vi "FTW-Regex-CapturingGroups.vi"(0 "Regex":refnum<data-value>, 11 "error in":errorcluster) -> (4 "Regex out":refnum<data-value>, 6 "Capture Groups":string[](array[string]), 15 "error out":errorcluster)   [LabVIEW 2014]
uses:
  core/FTW-Regex-Core-Structure.ctl
  error/FTW-ERR-ThrowError.vi
  error/FTW-ERR-NoErrorConstant.vi
  error/FTW-ERR-CallChain.vi
  string/FTW-STR-ReplaceWhitespace.vi
panel:
  # "Inputs"
  # "Outputs"
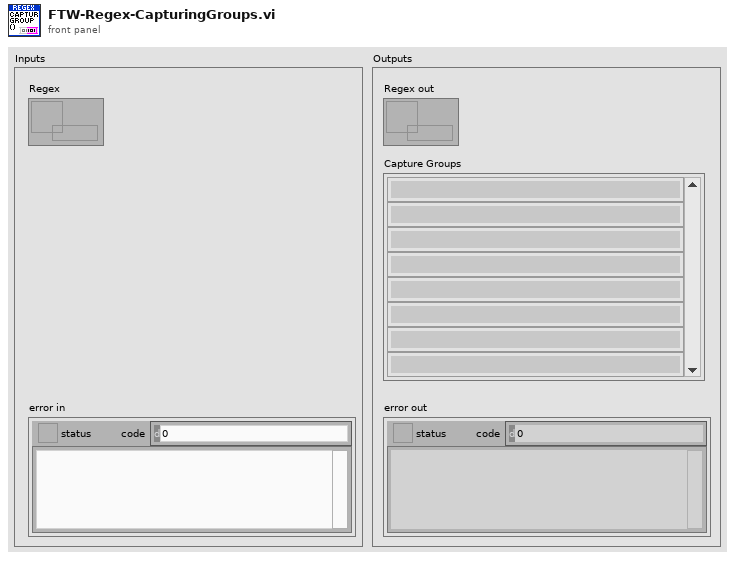
[diagram p1: front panel]
types:
  T1 = typedef "FTW-Regex-Core-Structure.ctl" = cluster{"Compiled Regex":u64}
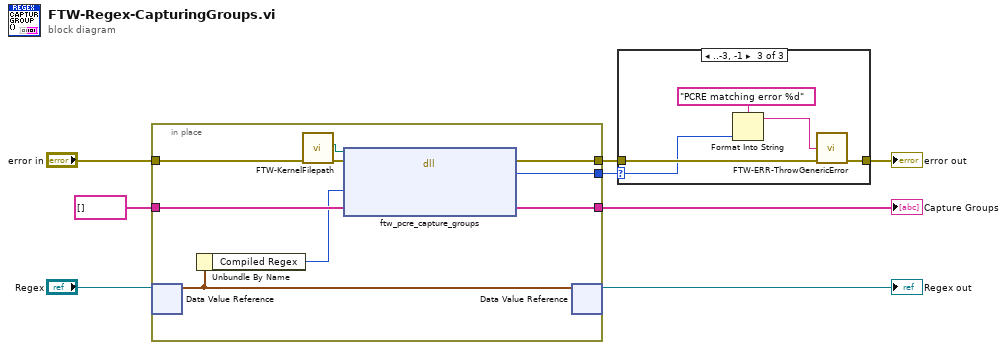
[diagram p0: block diagram]
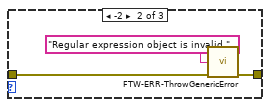
[diagram p3: hidden frame]
diagram:
  n1 = in-place {
    in-place-border: [w17] -> w5
    in-place-border: "error in" -> [w11]
    in-place-border: [w16] -> w7
    in-place-border: [w15] -> w4
    in-place-border: string[] [] -> [w14]
    n2 = in-place-dvr #1("Regex") -> (w13:T1)  [unwired: 1 out]
    n3 = Unbundle By Name(w13) -> ("Compiled Regex"=w12:u64)
    n4 = call "FTW-KernelFilepath.vi"("error in"=w11) -> ("error out"=w10:errorcluster, "Library Filepath"=w9:path)  [unwired: 8 in, 1 out]
    n5 = dll-call lib="?" fn="ftw_pcre_capture_groups"(path in=w9, error in=w10, "Compiled Regex"=w12, "Capture Groups"=w14) -> (error out=w17:errorcluster, "Return Value"=w16:i64, "Capture Groups"=w15:string[])  [unwired: 2 in, 1 out]
    n6 = in-place-dvr #1(w13) -> (→"Regex out":refnum<data-value>)  [unwired: 1 out]
  }
  "Capture Groups" <- w4
  n7 = case shown="..-3, -1" w7 {
    selector: w7 -> [_ _ w24]
    tunnel: [w18 w20 w25] -> w6
    tunnel: w5 -> [w18 w21 w26]
    frame 0.. {
    }
    frame -2 {
      n8 = call "FTW-ERR-ThrowGenericError.vi"("Error Message"="Regular expression object is invalid.", "error in"=w21) -> ("error out"=w20:errorcluster)  [unwired: 13 in]
    }
    frame ..-3, -1 {
      n9 = Format Into String(format string="PCRE matching error %d" ("Error Message"), w24) -> (resulting string=w23:string)  [unwired: 2 in, 1 out]
      n10 = call "FTW-ERR-ThrowGenericError.vi"("Error Message"=w23, "error in"=w26) -> ("error out"=w25:errorcluster)  [unwired: 13 in]
    }
  }
  "error out" <- w6
